vi "Subscribe to Results.vi"(8 "error in (no error)":errorcluster, 10 "Result Observer":refnum<class "Result Observer.lvclass">, 11 "LUnit Test Case In":refnum<class "LUnit Test Case.lvclass">) -> (0 "error out":errorcluster, 3 "LUnit Test Case Out":refnum<class "LUnit Test Case.lvclass">)   [LabVIEW 2020, in "LUnit Test Case.lvclass"]
uses:
  LUnit Test Case.lvclass
  Result Observer/Result Observer.lvclass
  LUnit Test Case.lvclass/LUnit Test Case.ctl
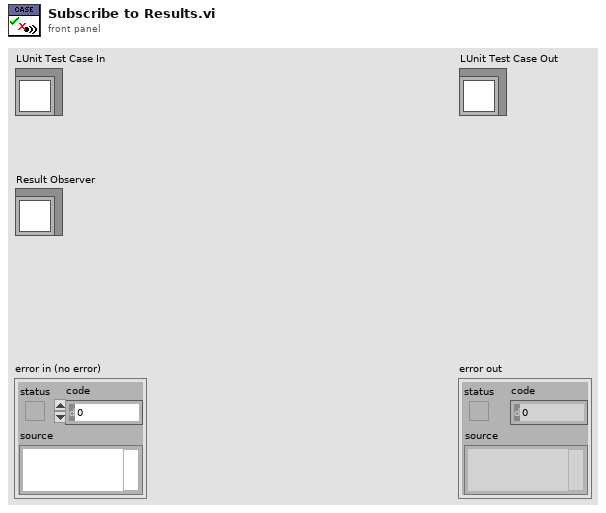
[diagram p1: front panel]
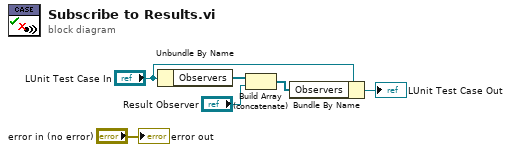
[diagram p0: block diagram]
diagram:
  n1 = Unbundle By Name("LUnit Test Case In") -> ("Observers"=w4:refnum<class "Result Observer.lvclass">[])
  n2 = Build Array (concatenate)(w4, "Result Observer") -> (w2:refnum<class "Result Observer.lvclass">[])
  n3 = Bundle By Name(cluster="LUnit Test Case In", "Observers"=w2) -> (→"LUnit Test Case Out":refnum<class "LUnit Test Case.lvclass">)
  "error out" <- "error in (no error)"
